vi "WavelengthControl_GetOutput.vi"(8 "error in (no error)":errorcluster, 11 "Topas":refnum<k24>) -> (0 "error out":errorcluster, 1 "WavelengthSettingCompletionPart":dbl, 2 "IsWavelengthSettingInProgress":bool, 3 "Topas Out":refnum<k24>, 5 "Interaction":string, 7 "Wavelength":dbl)   [LabVIEW 2017]
uses:
  D:/upwork/Laser Measurement Tool/Topas4PublicAPI/NET_SDK/Topas4Lib.dll
  Topas4PublicAPI/NET_SDK/Topas4Lib.dll
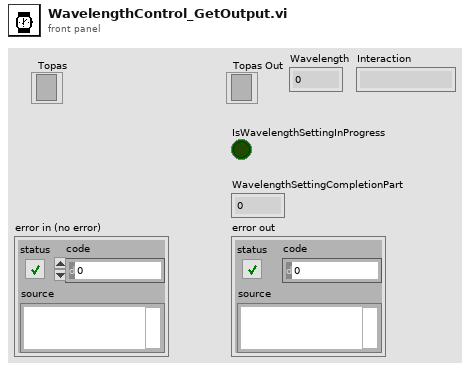
[diagram p1: front panel]
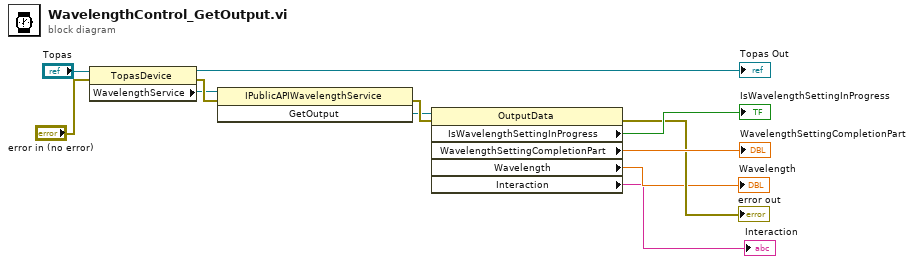
[diagram p0: block diagram]
diagram:
  n1 = property class="TopasDevice"(reference="Topas", error in="error in (no error)") -> (reference out=→"Topas Out":refnum<k24>, error out=w7:errorcluster, "WavelengthService"=w2:refnum<k24>)
  n2 = invoke class="IPublicAPIWavelengthService" method="GetOutput"(reference=w2, error in=w7) -> (error out=w6:errorcluster, "GetOutput"=w1:refnum<k24>)  [unwired: 1 in, 1 out]
  n3 = property class="OutputData"(reference=w1, error in=w6) -> (error out=→"error out":errorcluster, "IsWavelengthSettingInProgress"=→"IsWavelengthSettingInProgress":bool, "WavelengthSettingCompletionPart"=→"WavelengthSettingCompletionPart":dbl, "Wavelength"=→"Wavelength":dbl, "Interaction"=→"Interaction":string)  [unwired: 1 out]
